vi "_WriteTopData_TDMS_User_Data.vi"(8 "error in (no error)":errorcluster, 10 "Top Data in":T1={"Status"={"id_sensor"=0, "Ind."=FALSE, "sample time"=0, "rov_states"=enum."INIT", "acquisition_time"=timestamp(0 s since 1904-01-01), "modo_ctrl"=enum."Manual"}, "DAQ"={"id_daq"=0, "id_sensor"=0, "gps_"={"lat"=0.0, "lon"=0.0, "alt"=0.0}, "usbl_"={"x"=0.0, "y"=0.0, "z"=0.0}, "vess_ahrs_"={"pitch"=0.0, "roll"=0.0, "yaw"=0.0}, "acquisition_time"=timestamp(0 s since 1904-01-01)}, "User Data"={"id_sensor"=0, "id_daq"=0, "ci_habilitada"=FALSE, "acquisition_time"=timestamp(0 s since 1904-01-01), "CI Data"={"joy_1x"=0.0, "joy_1y"=0.0, "joy_1z"=0.0, "joy_1thumb"=0.0, "joy_1botIzq"=0, "joy_1botder"=0, "joy_1gatillo"=0, "modo_1bot"=0, "modo_2bot"=0, "modo_3bot"=0, "modo_4bot"=0, "pot"=0.0, "enc"=0.0, "joy_2x"=0.0, "joy_2y"=0.0, "joy_2z"=0.0, "joy_2bot"=0, "botella_1bot"=0, "botella_2bot"=0, "botella_3bot"=0, "botella_4bot"=0, "corer_1bot"=0, "corer_2bot"=0, "a_in"=0.0, "dio1"=0, "dio2"=0, "dio3"=0, "ci_acc_x"=0.0, "ci_acc_y"=0.0, "ci_acc_z"=0.0}, "Surface Data"={"modo_1ind"=0, "modo_2ind"=0, "modo_3ind"=0, "modo_4ind"=0, "botella_1ind"=0, "botella_2ind"=0, "botella_3ind"=0, "botella_4ind"=0, "corer_1ind"=0, "corer_2ind"=0, "lars_vel"=0.0, "lars_fwd"=0, "lars_rev"=0}}, "Virtual CI"={"id_sensor"=0, "id_daq"=0, "bus_260v"=FALSE, "m_6"=FALSE, "m_5"=FALSE, "m_2"=FALSE, "m_1"=FALSE, "m_4"=FALSE, "m_3"=FALSE, "luz_1"=FALSE, "luz_2"=FALSE, "luz_3"=FALSE, "pot_m1"=0.0, "pot_m2"=0.0, "pot_m3"=0.0, "pot_m4"=0.0, "pot_m5"=0.0, "pot_m6"=0.0, "pot_l1"=0.0, "pot_l2"=0.0, "pot_l3"=0.0, "pot_gen"=0.0, "fuente_muestras"=FALSE, "bot_1"=FALSE, "bot_2"=FALSE, "bot_3"=FALSE, "bot_4"=FALSE, "corer_1"=FALSE, "corer_2"=FALSE, "pot_c1"=0.0, "pot_c2"=0.0, "virtual_ci"=FALSE, "acquisition_time"=timestamp(0 s since 1904-01-01)}, "Control"={"depth_PID"={"Kp"=0.0, "Ti"=0.03, "Td"=0.001}, "heading_PID"={"Kp"=0.05, "Ti"=0.03, "Td"=0.001}, "altitude_PID"={"Kp"=0.05, "Ti"=0.03, "Td"=0.001}, "depth_sp"=0.0, "heading_sp"=0.0, "altitude_sp"=0.0, "m_PID_en"=FALSE, "PID_reset"=FALSE, "acquisition_time"=timestamp(0 s since 1904-01-01), "motor_PID"={"Kp"=0.05, "Ti"=0.03, "Td"=0.001}, "m1_lo"=0.0, "m1_hi"=0.0, "m1_en"=TRUE, "m2_lo"=0.0, "m2_hi"=0.0, "m2_en"=TRUE, "m3_lo"=0.0, "m3_hi"=0.0, "m3_en"=TRUE, "m4_lo"=0.0, "m4_hi"=5.0, "m4_en"=TRUE, "m5_lo"=-5.0, "m5_hi"=5.0, "m5_en"=TRUE, "m6_lo"=-5.0, "m6_hi"=5.0, "m6_en"=TRUE, "modo_ctrl"=enum."Manual"}} {"Virtual CI"."pot_c2" step=0.1; "Virtual CI"."pot_c1" step=0.01; "Virtual CI"."pot_gen" step=1.0; "Virtual CI"."pot_l3" step=0.01; "Virtual CI"."pot_l2" step=0.01; "Virtual CI"."pot_l1" step=0.01; "Virtual CI"."pot_m6" step=0.01; "Virtual CI"."pot_m5" step=0.01; "Virtual CI"."pot_m4" step=0.01; "Virtual CI"."pot_m3" step=0.01; "Virtual CI"."pot_m2" step=0.01; "Virtual CI"."pot_m1" step=0.01; "DAQ"."vess_ahrs_"."yaw" format="%.2g"; "DAQ"."vess_ahrs_"."roll" format="%.2g"; "DAQ"."vess_ahrs_"."pitch" format="%.2g"; "DAQ"."usbl_"."z" format="%.7g"; "DAQ"."usbl_"."y" format="%.7g"; "DAQ"."usbl_"."x" format="%.7g"; "DAQ"."gps_"."alt" format="%.7g"; "DAQ"."gps_"."lon" format="%.7g"; "DAQ"."gps_"."lat" format="%.7g"}, 11 "Refnum in":refnum<k34>) -> (0 "error out":errorcluster, 3 "Refnum out":refnum<k34>)   [LabVIEW 2018]
uses:
  TypeDefsTopside/Top Data.ctl
  Shared/Type Defs/ROV States.ctl
  TypeDefsSubsea/Modos Control.ctl
  TypeDefsTopside/DAQ Top Data.ctl
  TypeDefsTopside/User Data.ctl
  TypeDefsTopside/CI Data.ctl
  TypeDefsTopside/Surface Input Data.ctl
  TypeDefsTopside/Virtual User Interface Data.ctl
  TypeDefsTopside/Top Control.ctl
  TypeDefsSubsea/Type Defs Subsea.lvlib
  TypeDefsTopside/Type Defs Topside.lvlib
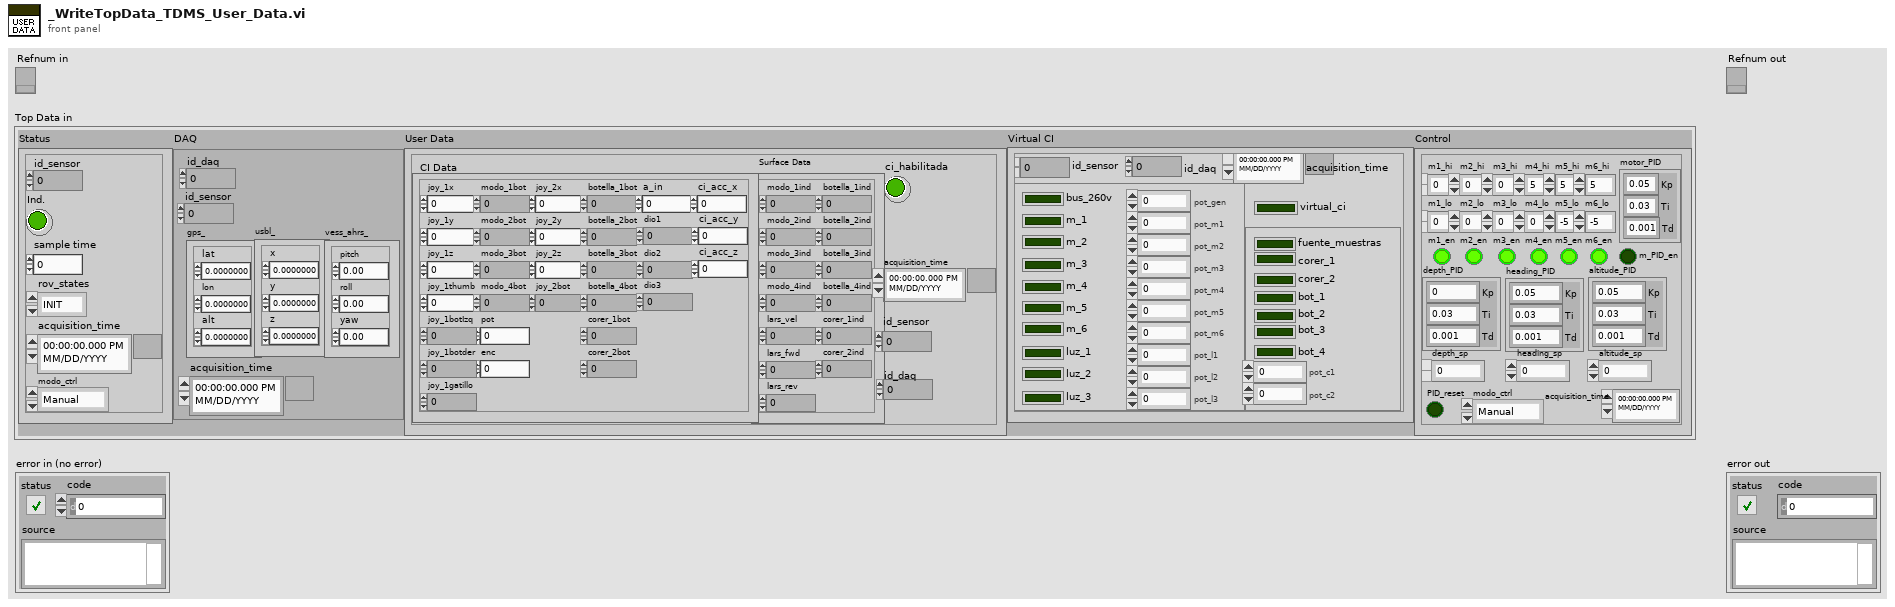
[diagram p1: front panel]
types:
  T1 = typedef "Type Defs Topside.lvlib/Top Data.ctl" = cluster{"Status":cluster{"id_sensor":u32, "Ind.":bool, "sample time":u32, "rov_states":T2, "acquisition_time":timestamp, "modo_ctrl":T3}, "DAQ":T4, "User Data":T5, "Virtual CI":T8, "Control":T9}
  T2 = typedef "Type Defs Subsea.lvlib/ROV States.ctl" = enum16{"INIT", "IDLE", "TEST", "RUN", "EMERGENCY", "EXIT"}
  T3 = typedef "Type Defs Subsea.lvlib/Modos Control.ctl" = enum16{"Manual", "Profundidad", "Altitud", "Rumbo", "P+R"}
  T4 = typedef "Type Defs Topside.lvlib/DAQ Top Data.ctl" = cluster{"id_daq":u32, "id_sensor":u32, "gps_":cluster{"lat":dbl, "lon":dbl, "alt":dbl}, "usbl_":cluster{"x":dbl, "y":dbl, "z":dbl}, "vess_ahrs_":cluster{"pitch":dbl, "roll":dbl, "yaw":dbl}, "acquisition_time":timestamp}
  T5 = typedef "Type Defs Topside.lvlib/User Data.ctl" = cluster{"id_sensor":u32, "id_daq":u64, "ci_habilitada":bool, "acquisition_time":timestamp, "CI Data":T6, "Surface Data":T7}
  T6 = typedef "Type Defs Topside.lvlib/CI Data.ctl" = cluster{"joy_1x":dbl, "joy_1y":dbl, "joy_1z":dbl, "joy_1thumb":dbl, "joy_1botIzq":u8, "joy_1botder":u8, "joy_1gatillo":u8, "modo_1bot":u8, "modo_2bot":u8, "modo_3bot":u8, "modo_4bot":u8, "pot":dbl, "enc":dbl, "joy_2x":dbl, "joy_2y":dbl, "joy_2z":dbl, "joy_2bot":u8, "botella_1bot":u8, "botella_2bot":u8, "botella_3bot":u8, "botella_4bot":u8, "corer_1bot":u8, "corer_2bot":u8, "a_in":dbl, "dio1":u8, "dio2":u8, "dio3":u8, "ci_acc_x":dbl, "ci_acc_y":dbl, "ci_acc_z":dbl}
  T7 = typedef "Type Defs Topside.lvlib/Surface Input Data.ctl" = cluster{"modo_1ind":u8, "modo_2ind":u8, "modo_3ind":u8, "modo_4ind":u8, "botella_1ind":u8, "botella_2ind":u8, "botella_3ind":u8, "botella_4ind":u8, "corer_1ind":u8, "corer_2ind":u8, "lars_vel":dbl, "lars_fwd":u8, "lars_rev":u8}
  T8 = typedef "Type Defs Topside.lvlib/Virtual User Interface Data.ctl" = cluster{"id_sensor":u32, "id_daq":u64, "bus_260v":bool, "m_6":bool, "m_5":bool, "m_2":bool, "m_1":bool, "m_4":bool, "m_3":bool, "luz_1":bool, "luz_2":bool, "luz_3":bool, "pot_m1":dbl, "pot_m2":dbl, "pot_m3":dbl, "pot_m4":dbl, "pot_m5":dbl, "pot_m6":dbl, "pot_l1":dbl, "pot_l2":dbl, "pot_l3":dbl, "pot_gen":dbl, "fuente_muestras":bool, "bot_1":bool, "bot_2":bool, "bot_3":bool, "bot_4":bool, "corer_1":bool, "corer_2":bool, "pot_c1":dbl, "pot_c2":dbl, "virtual_ci":bool, "acquisition_time":timestamp}
  T9 = typedef "Type Defs Topside.lvlib/Top Control.ctl" = cluster{"depth_PID":cluster{"Kp":dbl, "Ti":dbl, "Td":dbl}, "heading_PID":cluster{"Kp":dbl, "Ti":dbl, "Td":dbl}, "altitude_PID":cluster{"Kp":dbl, "Ti":dbl, "Td":dbl}, "depth_sp":dbl, "heading_sp":dbl, "altitude_sp":dbl, "m_PID_en":bool, "PID_reset":bool, "acquisition_time":timestamp, "motor_PID":cluster{"Kp":dbl, "Ti":dbl, "Td":dbl}, "m1_lo":dbl, "m1_hi":dbl, "m1_en":bool, "m2_lo":dbl, "m2_hi":dbl, "m2_en":bool, "m3_lo":dbl, "m3_hi":dbl, "m3_en":bool, "m4_lo":dbl, "m4_hi":dbl, "m4_en":bool, "m5_lo":dbl, "m5_hi":dbl, "m5_en":bool, "m6_lo":dbl, "m6_hi":dbl, "m6_en":bool, "modo_ctrl":T3}
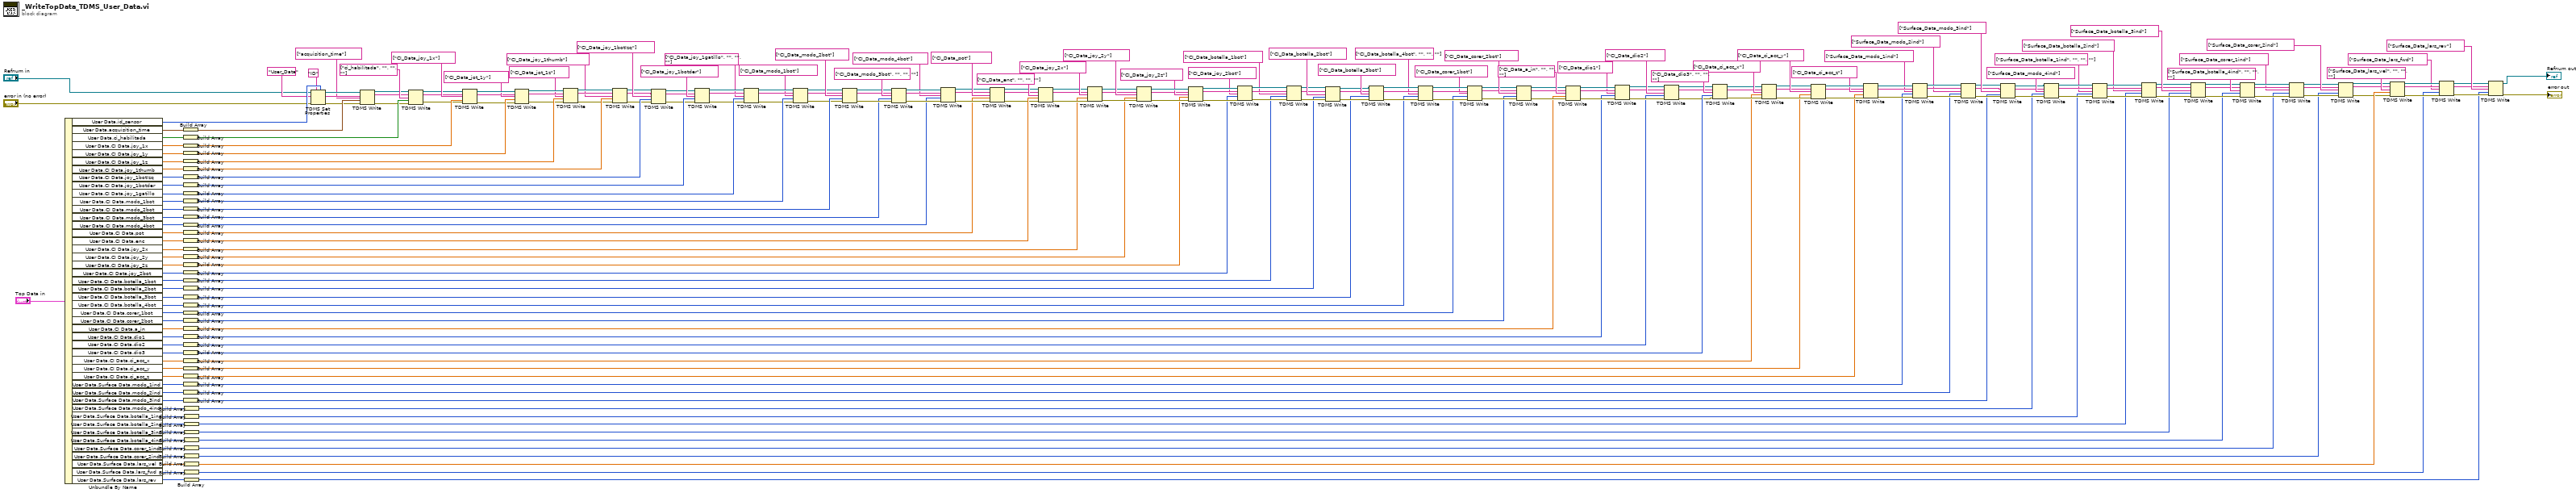
[diagram p0: block diagram]
diagram:
  n1 = Unbundle By Name("Top Data in") -> ("User Data.id_sensor"=w266:u32, "User Data.acquisition_time"=w267:timestamp, "User Data.ci_habilitada"=w206:bool, "User Data.CI Data.joy_1x"=w205:dbl, "User Data.CI Data.joy_1y"=w204:dbl, "User Data.CI Data.joy_1z"=w203:dbl, "User Data.CI Data.joy_1thumb"=w202:dbl, "User Data.CI Data.joy_1botIzq"=w201:u8, "User Data.CI Data.joy_1botder"=w200:u8, "User Data.CI Data.joy_1gatillo"=w199:u8, "User Data.CI Data.modo_1bot"=w198:u8, "User Data.CI Data.modo_2bot"=w197:u8, "User Data.CI Data.modo_3bot"=w196:u8, "User Data.CI Data.modo_4bot"=w195:u8, "User Data.CI Data.pot"=w194:dbl, "User Data.CI Data.enc"=w87:dbl, "User Data.CI Data.joy_2x"=w86:dbl, "User Data.CI Data.joy_2y"=w85:dbl, "User Data.CI Data.joy_2z"=w84:dbl, "User Data.CI Data.joy_2bot"=w83:u8, "User Data.CI Data.botella_1bot"=w82:u8, "User Data.CI Data.botella_2bot"=w81:u8, "User Data.CI Data.botella_3bot"=w80:u8, "User Data.CI Data.botella_4bot"=w79:u8, "User Data.CI Data.corer_1bot"=w78:u8, "User Data.CI Data.corer_2bot"=w77:u8, "User Data.CI Data.a_in"=w76:dbl, "User Data.CI Data.dio1"=w75:u8, "User Data.CI Data.dio2"=w74:u8, "User Data.CI Data.dio3"=w73:u8, "User Data.CI Data.ci_acc_x"=w72:dbl, "User Data.CI Data.ci_acc_y"=w71:dbl, "User Data.CI Data.ci_acc_z"=w70:dbl, "User Data.Surface Data.modo_1ind"=w69:u8, "User Data.Surface Data.modo_2ind"=w68:u8, "User Data.Surface Data.modo_3ind"=w67:u8, "User Data.Surface Data.modo_4ind"=w66:u8, "User Data.Surface Data.botella_1ind"=w65:u8, "User Data.Surface Data.botella_2ind"=w64:u8, "User Data.Surface Data.botella_3ind"=w63:u8, "User Data.Surface Data.botella_4ind"=w62:u8, "User Data.Surface Data.corer_1ind"=w61:u8, "User Data.Surface Data.corer_2ind"=w60:u8, "User Data.Surface Data.lars_vel"=w59:dbl, "User Data.Surface Data.lars_fwd"=w58:u8, "User Data.Surface Data.lars_rev"=w57:u8)
  n2 = Build Array(w267) -> (w268:timestamp[])
  n3 = Build Array(w206) -> (w269:bool[])
  n4 = Build Array(w205) -> (w270:dbl[])
  n5 = Build Array(w204) -> (w271:dbl[])
  n6 = Build Array(w203) -> (w272:dbl[])
  n7 = Build Array(w202) -> (w273:dbl[])
  n8 = Build Array(w201) -> (w274:u8[])
  n9 = Build Array(w200) -> (w275:u8[])
  n10 = Build Array(w199) -> (w276:u8[])
  n11 = Build Array(w198) -> (w277:u8[])
  n12 = Build Array(w197) -> (w278:u8[])
  n13 = Build Array(w196) -> (w215:u8[])
  n14 = Build Array(w195) -> (w214:u8[])
  n15 = Build Array(w194) -> (w213:dbl[])
  n16 = Build Array(w87) -> (w56:dbl[])
  n17 = Build Array(w86) -> (w55:dbl[])
  n18 = Build Array(w85) -> (w54:dbl[])
  n19 = Build Array(w84) -> (w53:dbl[])
  n20 = Build Array(w83) -> (w52:u8[])
  n21 = Build Array(w82) -> (w51:u8[])
  n22 = Build Array(w81) -> (w50:u8[])
  n23 = Build Array(w80) -> (w49:u8[])
  n24 = Build Array(w79) -> (w48:u8[])
  n25 = Build Array(w78) -> (w47:u8[])
  n26 = Build Array(w77) -> (w46:u8[])
  n27 = Build Array(w76) -> (w45:dbl[])
  n28 = Build Array(w75) -> (w44:u8[])
  n29 = Build Array(w74) -> (w43:u8[])
  n30 = Build Array(w73) -> (w42:u8[])
  n31 = Build Array(w72) -> (w32:dbl[])
  n32 = Build Array(w71) -> (w31:dbl[])
  n33 = Build Array(w70) -> (w30:dbl[])
  n34 = Build Array(w69) -> (w29:u8[])
  n35 = Build Array(w68) -> (w28:u8[])
  n36 = Build Array(w67) -> (w27:u8[])
  n37 = Build Array(w66) -> (w26:u8[])
  n38 = Build Array(w65) -> (w25:u8[])
  n39 = Build Array(w64) -> (w24:u8[])
  n40 = Build Array(w63) -> (w23:u8[])
  n41 = Build Array(w62) -> (w22:u8[])
  n42 = Build Array(w61) -> (w21:u8[])
  n43 = Build Array(w60) -> (w20:u8[])
  n44 = Build Array(w59) -> (w19:dbl[])
  n45 = Build Array(w58) -> (w18:u8[])
  n46 = Build Array(w57) -> (w17:u8[])
  n47 = TDMS Set Properties(5:w266, 7:"ID" ("property names"), 8:"error in (no error)", 10:"User_Data" ("group name in (Untitled)"), 11:"Refnum in") -> (0:w236:errorcluster, 2:w235:string, 3:w233:refnum<k34>)  [unwired: 1 in, 1 out]
  n48 = TDMS Write(0:w233, 5:w235, 7:string[] ["acquisition_time"] ("channel name(s) in (Untitled)"), 9:w268, 11:w236) -> (4:w229:refnum<k34>, 6:w228:string, 15:w230:errorcluster)  [unwired: 1 in, 1 out]
  n49 = TDMS Write(0:w229, 5:w228, 7:string[] ["ci_habilitada", "", "", ""] ("channel name(s) in (Untitled)"), 9:w269, 11:w230) -> (4:w3:refnum<k34>, 6:w2:string, 15:w1:errorcluster)  [unwired: 1 in, 1 out]
  n50 = TDMS Write(0:w3, 5:w2, 7:string[] ["CI_Data_joy_1x"] ("channel name(s) in (Untitled)"), 9:w270, 11:w1) -> (4:w211:refnum<k34>, 6:w209:string, 15:w212:errorcluster)  [unwired: 1 in, 1 out]
  n51 = TDMS Write(0:w211, 5:w209, 7:string[] ["CI_Data_jot_1y"] ("channel name(s) in (Untitled)"), 9:w271, 11:w212) -> (4:w241:refnum<k34>, 6:w242:string, 15:w240:errorcluster)  [unwired: 1 in, 1 out]
  n52 = TDMS Write(0:w241, 5:w242, 7:string[] ["CI_Data_jot_1z"] ("channel name(s) in (Untitled)"), 9:w272, 11:w240) -> (4:w244:refnum<k34>, 6:w245:string, 15:w243:errorcluster)  [unwired: 1 in, 1 out]
  n53 = TDMS Write(0:w244, 5:w245, 7:string[] ["CI_Data_joy_1thumb"] ("channel name(s) in (Untitled)"), 9:w273, 11:w243) -> (4:w260:refnum<k34>, 6:w262:string, 15:w261:errorcluster)  [unwired: 1 in, 1 out]
  n54 = TDMS Write(0:w260, 5:w262, 7:string[] ["CI_Data_joy_1botIzq"] ("channel name(s) in (Untitled)"), 9:w274, 11:w261) -> (4:w257:refnum<k34>, 6:w258:string, 15:w263:errorcluster)  [unwired: 1 in, 1 out]
  n55 = TDMS Write(0:w257, 5:w258, 7:string[] ["CI_Data_joy_1botder"] ("channel name(s) in (Untitled)"), 9:w275, 11:w263) -> (4:w255:refnum<k34>, 6:w256:string, 15:w254:errorcluster)  [unwired: 1 in, 1 out]
  n56 = TDMS Write(0:w255, 5:w256, 7:string[] ["CI_Data_joy_1gatillo", "", "", ""] ("channel name(s) in (Untitled)"), 9:w276, 11:w254) -> (4:w248:refnum<k34>, 6:w249:string, 15:w247:errorcluster)  [unwired: 1 in, 1 out]
  n57 = TDMS Write(0:w248, 5:w249, 7:string[] ["CI_Data_modo_1bot"] ("channel name(s) in (Untitled)"), 9:w277, 11:w247) -> (4:w251:refnum<k34>, 6:w252:string, 15:w250:errorcluster)  [unwired: 1 in, 1 out]
  n58 = TDMS Write(0:w251, 5:w252, 7:string[] ["CI_Data_modo_2bot"] ("channel name(s) in (Untitled)"), 9:w278, 11:w250) -> (4:w217:refnum<k34>, 6:w208:string, 15:w216:errorcluster)  [unwired: 1 in, 1 out]
  n59 = TDMS Write(0:w217, 5:w208, 7:string[] ["CI_Data_modo_3bot", "", "", ""] ("channel name(s) in (Untitled)"), 9:w215, 11:w216) -> (4:w220:refnum<k34>, 6:w221:string, 15:w219:errorcluster)  [unwired: 1 in, 1 out]
  n60 = TDMS Write(0:w220, 5:w221, 7:string[] ["CI_Data_modo_4bot"] ("channel name(s) in (Untitled)"), 9:w214, 11:w219) -> (4:w223:refnum<k34>, 6:w224:string, 15:w222:errorcluster)  [unwired: 1 in, 1 out]
  n61 = TDMS Write(0:w223, 5:w224, 7:string[] ["CI_Data_pot"] ("channel name(s) in (Untitled)"), 9:w213, 11:w222) -> (4:w10:refnum<k34>, 6:w6:string, 15:w9:errorcluster)  [unwired: 1 in, 1 out]
  n62 = TDMS Write(0:w10, 5:w6, 7:string[] ["CI_Data_enc", "", "", ""] ("channel name(s) in (Untitled)"), 9:w56, 11:w9) -> (4:w162:refnum<k34>, 6:w161:string, 15:w163:errorcluster)  [unwired: 1 in, 1 out]
  n63 = TDMS Write(0:w162, 5:w161, 7:string[] ["CI_Data_joy_2x"] ("channel name(s) in (Untitled)"), 9:w55, 11:w163) -> (4:w159:refnum<k34>, 6:w158:string, 15:w160:errorcluster)  [unwired: 1 in, 1 out]
  n64 = TDMS Write(0:w159, 5:w158, 7:string[] ["CI_Data_joy_2y"] ("channel name(s) in (Untitled)"), 9:w54, 11:w160) -> (4:w144:refnum<k34>, 6:w142:string, 15:w145:errorcluster)  [unwired: 1 in, 1 out]
  n65 = TDMS Write(0:w144, 5:w142, 7:string[] ["CI_Data_joy_2z"] ("channel name(s) in (Untitled)"), 9:w53, 11:w145) -> (4:w169:refnum<k34>, 6:w170:string, 15:w168:errorcluster)  [unwired: 1 in, 1 out]
  n66 = TDMS Write(0:w169, 5:w170, 7:string[] ["CI_Data_joy_2bot"] ("channel name(s) in (Untitled)"), 9:w52, 11:w168) -> (4:w172:refnum<k34>, 6:w173:string, 15:w171:errorcluster)  [unwired: 1 in, 1 out]
  n67 = TDMS Write(0:w172, 5:w173, 7:string[] ["CI_Data_botella_1bot"] ("channel name(s) in (Untitled)"), 9:w51, 11:w171) -> (4:w188:refnum<k34>, 6:w190:string, 15:w189:errorcluster)  [unwired: 1 in, 1 out]
  n68 = TDMS Write(0:w188, 5:w190, 7:string[] ["CI_Data_botella_2bot"] ("channel name(s) in (Untitled)"), 9:w50, 11:w189) -> (4:w185:refnum<k34>, 6:w186:string, 15:w191:errorcluster)  [unwired: 1 in, 1 out]
  n69 = TDMS Write(0:w185, 5:w186, 7:string[] ["CI_Data_botella_3bot"] ("channel name(s) in (Untitled)"), 9:w49, 11:w191) -> (4:w183:refnum<k34>, 6:w184:string, 15:w182:errorcluster)  [unwired: 1 in, 1 out]
  n70 = TDMS Write(0:w183, 5:w184, 7:string[] ["CI_Data_botella_4bot", "", "", ""] ("channel name(s) in (Untitled)"), 9:w48, 11:w182) -> (4:w176:refnum<k34>, 6:w177:string, 15:w175:errorcluster)  [unwired: 1 in, 1 out]
  n71 = TDMS Write(0:w176, 5:w177, 7:string[] ["CI_Data_corer_1bot"] ("channel name(s) in (Untitled)"), 9:w47, 11:w175) -> (4:w179:refnum<k34>, 6:w180:string, 15:w178:errorcluster)  [unwired: 1 in, 1 out]
  n72 = TDMS Write(0:w179, 5:w180, 7:string[] ["CI_Data_corer_2bot"] ("channel name(s) in (Untitled)"), 9:w46, 11:w178) -> (4:w147:refnum<k34>, 6:w141:string, 15:w146:errorcluster)  [unwired: 1 in, 1 out]
  n73 = TDMS Write(0:w147, 5:w141, 7:string[] ["CI_Data_a_in", "", "", ""] ("channel name(s) in (Untitled)"), 9:w45, 11:w146) -> (4:w150:refnum<k34>, 6:w151:string, 15:w149:errorcluster)  [unwired: 1 in, 1 out]
  n74 = TDMS Write(0:w150, 5:w151, 7:string[] ["CI_Data_dio1"] ("channel name(s) in (Untitled)"), 9:w44, 11:w149) -> (4:w153:refnum<k34>, 6:w154:string, 15:w152:errorcluster)  [unwired: 1 in, 1 out]
  n75 = TDMS Write(0:w153, 5:w154, 7:string[] ["CI_Data_dio2"] ("channel name(s) in (Untitled)"), 9:w43, 11:w152) -> (4:w13:refnum<k34>, 6:w5:string, 15:w14:errorcluster)  [unwired: 1 in, 1 out]
  n76 = TDMS Write(0:w13, 5:w5, 7:string[] ["CI_Data_dio3", "", "", ""] ("channel name(s) in (Untitled)"), 9:w42, 11:w14) -> (4:w109:refnum<k34>, 6:w108:string, 15:w110:errorcluster)  [unwired: 1 in, 1 out]
  n77 = TDMS Write(0:w109, 5:w108, 7:string[] ["CI_Data_ci_acc_x"] ("channel name(s) in (Untitled)"), 9:w32, 11:w110) -> (4:w106:refnum<k34>, 6:w105:string, 15:w107:errorcluster)  [unwired: 1 in, 1 out]
  n78 = TDMS Write(0:w106, 5:w105, 7:string[] ["CI_Data_ci_acc_y"] ("channel name(s) in (Untitled)"), 9:w31, 11:w107) -> (4:w91:refnum<k34>, 6:w89:string, 15:w92:errorcluster)  [unwired: 1 in, 1 out]
  n79 = TDMS Write(0:w91, 5:w89, 7:string[] ["CI_Data_ci_acc_z"] ("channel name(s) in (Untitled)"), 9:w30, 11:w92) -> (4:w116:refnum<k34>, 6:w117:string, 15:w115:errorcluster)  [unwired: 1 in, 1 out]
  n80 = TDMS Write(0:w116, 5:w117, 7:string[] ["Surface_Data_modo_1ind"] ("channel name(s) in (Untitled)"), 9:w29, 11:w115) -> (4:w119:refnum<k34>, 6:w120:string, 15:w118:errorcluster)  [unwired: 1 in, 1 out]
  n81 = TDMS Write(0:w119, 5:w120, 7:string[] ["Surface_Data_modo_2ind"] ("channel name(s) in (Untitled)"), 9:w28, 11:w118) -> (4:w135:refnum<k34>, 6:w137:string, 15:w136:errorcluster)  [unwired: 1 in, 1 out]
  n82 = TDMS Write(0:w135, 5:w137, 7:string[] ["Surface_Data_modo_3ind"] ("channel name(s) in (Untitled)"), 9:w27, 11:w136) -> (4:w132:refnum<k34>, 6:w133:string, 15:w138:errorcluster)  [unwired: 1 in, 1 out]
  n83 = TDMS Write(0:w132, 5:w133, 7:string[] ["Surface_Data_modo_4ind"] ("channel name(s) in (Untitled)"), 9:w26, 11:w138) -> (4:w130:refnum<k34>, 6:w131:string, 15:w129:errorcluster)  [unwired: 1 in, 1 out]
  n84 = TDMS Write(0:w130, 5:w131, 7:string[] ["Surface_Data_botella_1ind", "", "", ""] ("channel name(s) in (Untitled)"), 9:w25, 11:w129) -> (4:w123:refnum<k34>, 6:w124:string, 15:w122:errorcluster)  [unwired: 1 in, 1 out]
  n85 = TDMS Write(0:w123, 5:w124, 7:string[] ["Surface_Data_botella_2ind"] ("channel name(s) in (Untitled)"), 9:w24, 11:w122) -> (4:w126:refnum<k34>, 6:w127:string, 15:w125:errorcluster)  [unwired: 1 in, 1 out]
  n86 = TDMS Write(0:w126, 5:w127, 7:string[] ["Surface_Data_botella_3ind"] ("channel name(s) in (Untitled)"), 9:w23, 11:w125) -> (4:w94:refnum<k34>, 6:w88:string, 15:w93:errorcluster)  [unwired: 1 in, 1 out]
  n87 = TDMS Write(0:w94, 5:w88, 7:string[] ["Surface_Data_botella_4ind", "", "", ""] ("channel name(s) in (Untitled)"), 9:w22, 11:w93) -> (4:w97:refnum<k34>, 6:w98:string, 15:w96:errorcluster)  [unwired: 1 in, 1 out]
  n88 = TDMS Write(0:w97, 5:w98, 7:string[] ["Surface_Data_corer_1ind"] ("channel name(s) in (Untitled)"), 9:w21, 11:w96) -> (4:w100:refnum<k34>, 6:w101:string, 15:w99:errorcluster)  [unwired: 1 in, 1 out]
  n89 = TDMS Write(0:w100, 5:w101, 7:string[] ["Surface_Data_corer_2ind"] ("channel name(s) in (Untitled)"), 9:w20, 11:w99) -> (4:w16:refnum<k34>, 6:w4:string, 15:w15:errorcluster)  [unwired: 1 in, 1 out]
  n90 = TDMS Write(0:w16, 5:w4, 7:string[] ["Surface_Data_lars_vel", "", "", ""] ("channel name(s) in (Untitled)"), 9:w19, 11:w15) -> (4:w35:refnum<k34>, 6:w36:string, 15:w34:errorcluster)  [unwired: 1 in, 1 out]
  n91 = TDMS Write(0:w35, 5:w36, 7:string[] ["Surface_Data_lars_fwd"] ("channel name(s) in (Untitled)"), 9:w18, 11:w34) -> (4:w38:refnum<k34>, 6:w39:string, 15:w37:errorcluster)  [unwired: 1 in, 1 out]
  n92 = TDMS Write(0:w38, 5:w39, 7:string[] ["Surface_Data_lars_rev"] ("channel name(s) in (Untitled)"), 9:w17, 11:w37) -> (4:→"Refnum out":refnum<k34>, 15:→"error out":errorcluster)  [unwired: 1 in, 2 out]
